vi "EV3Tests.vi"() -> ()   [LabVIEW 2016]
uses:
  VIs/uPythonX/uPythonX.xctl
panel:
  in  "Sound and Light":T1(xcontrol)={"VISA Refnum in"="169.254.29.229", "All Code"="#!/usr/bin/env pybricks-micropython\n\nfrom pybricks import ev3brick as brick\nfrom pybricks.parameters import Button, Color,ImageFile\nfrom pybricks.tools import print, wait\n\n# Write your program here\n# A high pitch (1500 Hz) for one second (1000 ms) at 50% volume\nbrick.sound.beep(500, 1000, 20)\n\nbrick.light(Color.RED)\nLight = [Color.BLACK, Color.GREEN, Color.YELLOW, Color.RED, Color.ORANGE]\n\nfor color in Light:\n    print(color)\n    try:\n        brick.light(color)\n    except:\n        print('bad')\n    wait(500)\n\nbrick.display.clear()\nbrick.display.text(brick.battery.voltage(), (0, 50))\nwhile not Button.CENTER in brick.buttons():\n    wait(100)\nbrick.display.image(ImageFile.UP)\nwhile not Button.CENTER in brick.buttons():\n    wait(100)\n\nwhile True:\n    # Do something if the left button is pressed\n    if Button.LEFT in brick.buttons():\n        print(\"The left button is pressed.\")\n        break\n    wait(100)"}
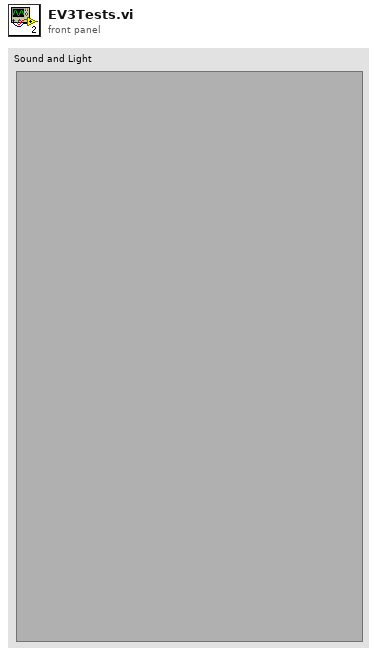
[diagram p1: front panel]
types:
  T1 = cluster{"VISA Refnum in":refnum<visa-resource-name>, "All Code":string}
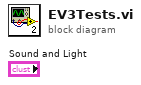
[diagram p0: block diagram]
diagram:
